vi "Write PNG File with Alpha.vi"(8 "error in (no error)":errorcluster, 10 ".png Filepath":path, 11 "ARGB Image Source":T1) -> (0 "error out":errorcluster, 3 ".png Filepath (duplicate)":path)   [LabVIEW 2020, in "g_ar_toolkit.image.lvlib"]
uses:
  g_ar_toolkit.image.lvlib
  ARGB Image.ctl
  9723f547-2605-4a38-b7b5-a8bc0a93fff0.vi
  g_ar_toolkit.common/Module Path.vi
  <vilib>/Utility/error.llb/Error Cluster From Error Code.vi
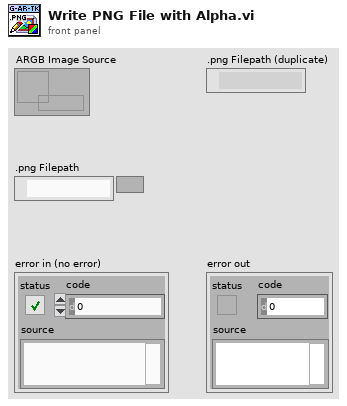
[diagram p1: front panel]
types:
  T1 = typedef "g_ar_toolkit.image.lvlib/ARGB Image.ctl" = refnum<data-value>
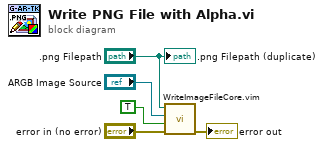
[diagram p0: block diagram]
diagram:
  n1 = call "WriteImageFileCore.vim"("error in (no error)"="error in (no error)", "SaveAlpha"=TRUE, "Src"="ARGB Image Source", "Filepath"=".png Filepath") -> ("error out"=→"error out":errorcluster)  [unwired: 7 in]
  ".png Filepath (duplicate)" <- ".png Filepath"
